vi "GetClassTemplates.vi"(0 "ClassWriterGOOP300 in":refnum<class "ClassWriterGOOP300.lvclass">, 1 "DerivedFromThisClass(if any)":refnum<vi>, 5 "error in (no error)":errorcluster) -> (14 "ClassWriterGOOP300 out":refnum<class "ClassWriterGOOP300.lvclass">, 15 "Templates":T1[](array[typedef]), 19 "error out":errorcluster)   [LabVIEW 2016, in "ClassWriterGOOP300.lvclass"]
uses:
  <resource>/Framework/Providers/Open_GDS/ClassProviders/Provider_EndevoGOOP300/ClassWriterGOOP300_class/ClassWriterGOOP300.lvclass
  <resource>/Framework/Providers/Open_GDS/ClassProviders/Provider_BaseClassInterface/ClassTemplateType.ctl
  <resource>/Framework/Providers/Open_GDS/ClassProviders/Provider_EndevoGOOP300/Templates/EndevoTemplateNames.ctl
  <resource>/Framework/Providers/Open_GDS/ClassProviders/Common/ScriptingFunctions/Scripting_ConnectorPanePatternType.ctl
  <resource>/Framework/Providers/Open_GDS/ClassProviders/Provider_BaseClassInterface/ClassWriter_class/ClassWriter.lvclass
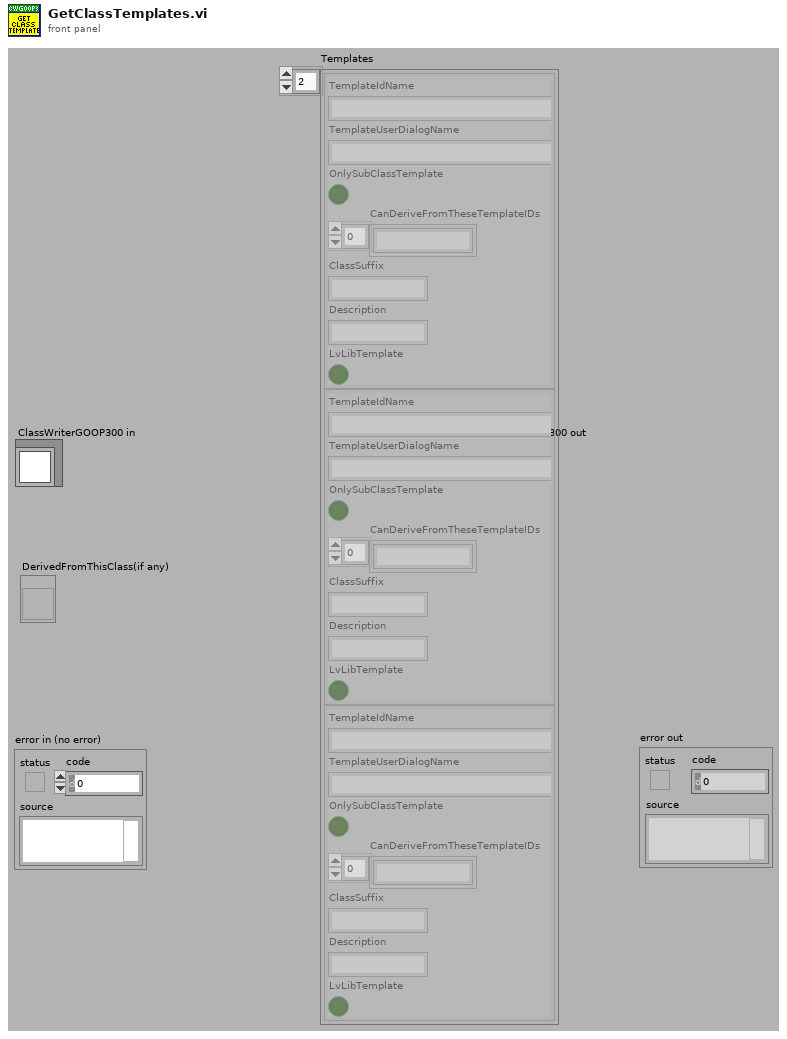
[diagram p1: front panel]
types:
  T1 = typedef "ClassWriter.lvclass/ClassTemplateType.ctl" = cluster{"TemplateIdName":string, "TemplateUserDialogName":string, "OnlySubClassTemplate":bool, "CanDeriveFromTheseTemplateIDs":string[], "ClassSuffix":string, "Description":string, "LvLibTemplate":bool}
  T2 = typedef "EndevoTemplateNames.ctl" = enum16{"BaseTemplate", "SubTemplate", "BaseTemplate_4x4x4", "SubTemplate_4x4x4", "SingletonTemplate"}
  T3 = typedef "Scripting_ConnectorPanePatternType.ctl" = u16
  T4 = typedef "GDSLvCLass_ClassSettingsType.ctl" = cluster{"ClassProviderName":string, "ClassTemplateUsed":string, "ClassTemplateVersion":string, "ClassDescription":string, "PlugIns":T5[], "ConnectorPanePattern":string}
  T5 = typedef "GDSLvClass_PlugIn.ctl" = cluster{"Type":T6, "ID":string, "Version":string, "Path":path, "Name":string, "Data":variant}
  T6 = typedef "GDSLvClass_PlugInTypes.ctl" = enum16{"DesignPattern", "MethodTypes"}
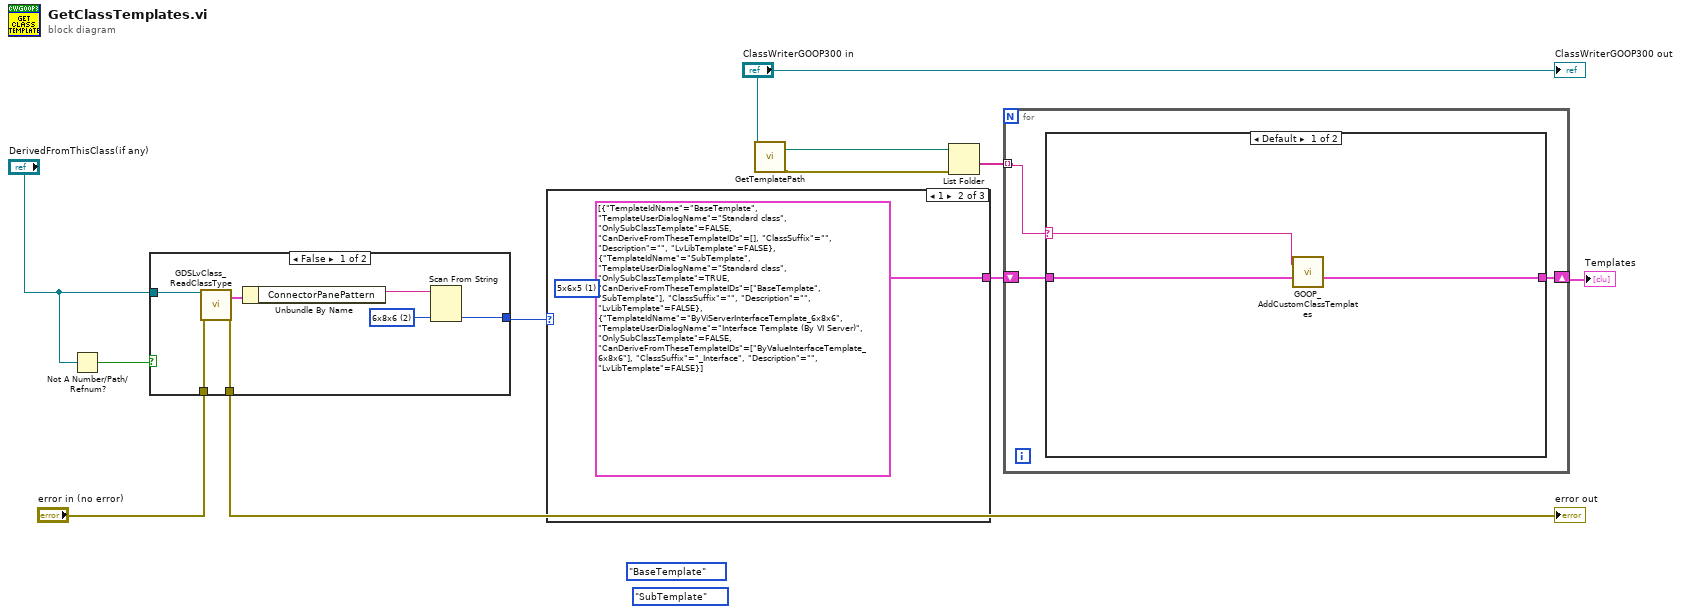
[diagram p0: block diagram]
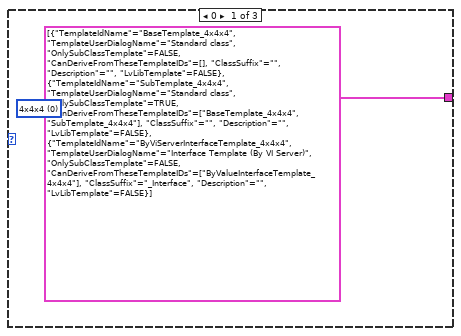
[diagram p2: hidden frame]
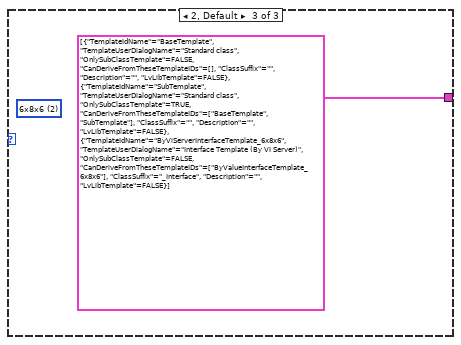
[diagram p3: hidden frame]
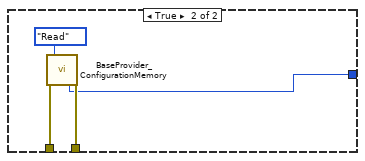
[diagram p4: hidden frame]
diagram:
  (unwired) EndevoTemplateNames."BaseTemplate" ("TemplateNames")
  (unwired) EndevoTemplateNames."SubTemplate" ("TemplateNames")
  n1 = Not A Number/Path/Refnum?(number/path/refnum="DerivedFromThisClass(if any)") -> (NaN/Path/Refnum?=w5:bool)
  n2 = case shown="False" w5 {
    tunnel: "error in (no error)" -> [w15 w21]
    tunnel: "DerivedFromThisClass(if any)" -> [w14 _]
    tunnel: [w13 w20] -> w1
    tunnel: [w12 w19] -> w4
    frame False {
      w16 = T3 2 items=["4x4x4", "5x6x5", "6x8x6"] ("Pattern")
      n3 = call <resource>:"GDSLvClass_ReadClassType.vi"("Class Refnum In"=w14, "error in (no error)"=w15) -> ("ClassSettings"=w18:T4, "error out"=w13:errorcluster)  [unwired: 15 in, 1 out]
      n4 = Unbundle By Name(w18) -> ("ConnectorPanePattern"=w17:string)
      n5 = Scan From String(input string=w17, default 1=w16) -> (output 1=w12:T3)  [unwired: 3 in, 3 out]
    }
    frame True {
      n6 = call <resource>:"BaseProvider_ConfigurationMemory.vi"("error in (no error)"=w21, "Action"=enum16{"Read", "Load", "Save"}."Read") -> ("PatternOut"=w19:T3, "error out"=w20:errorcluster)  [unwired: 11 in, 5 out]
    }
  }
  "error out" <- w1
  n7 = case shown="1" w4 {
    tunnel: [T1[] [{"TemplateIdName"="BaseTemplate_4x4x4", "TemplateUserDialogName"="Standard class", "OnlySubClassTemplate"=FALSE, "CanDeriveFromTheseTemplateIDs"=[], "ClassSuffix"="", "Description"="", "LvLibTemplate"=FALSE}, {"TemplateIdName"="SubTemplate_4x4x4", "TemplateUserDialogName"="Standard class", "OnlySubClassTemplate"=TRUE, "CanDeriveFromTheseTemplateIDs"=["BaseTemplate_4x4x4", "SubTemplate_4x4x4"], "ClassSuffix"="", "Description"="", "LvLibTemplate"=FALSE}, {"TemplateIdName"="ByViServerInterfaceTemplate_4x4x4", "TemplateUserDialogName"="Interface Template (By VI Server)", "OnlySubClassTemplate"=FALSE, "CanDeriveFromTheseTemplateIDs"=["ByValueInterfaceTemplate_4x4x4"], "ClassSuffix"="_Interface", "Description"="", "LvLibTemplate"=FALSE}] ("TemplateIdNames") T1[] [{"TemplateIdName"="BaseTemplate", "TemplateUserDialogName"="Standard class", "OnlySubClassTemplate"=FALSE, "CanDeriveFromTheseTemplateIDs"=[], "ClassSuffix"="", "Description"="", "LvLibTemplate"=FALSE}, {"TemplateIdName"="SubTemplate", "TemplateUserDialogName"="Standard class", "OnlySubClassTemplate"=TRUE, "CanDeriveFromTheseTemplateIDs"=["BaseTemplate", "SubTemplate"], "ClassSuffix"="", "Description"="", "LvLibTemplate"=FALSE}, {"TemplateIdName"="ByViServerInterfaceTemplate_6x8x6", "TemplateUserDialogName"="Interface Template (By VI Server)", "OnlySubClassTemplate"=FALSE, "CanDeriveFromTheseTemplateIDs"=["ByValueInterfaceTemplate_6x8x6"], "ClassSuffix"="_Interface", "Description"="", "LvLibTemplate"=FALSE}] ("TemplateIdNames") T1[] [{"TemplateIdName"="BaseTemplate", "TemplateUserDialogName"="Standard class", "OnlySubClassTemplate"=FALSE, "CanDeriveFromTheseTemplateIDs"=[], "ClassSuffix"="", "Description"="", "LvLibTemplate"=FALSE}, {"TemplateIdName"="SubTemplate", "TemplateUserDialogName"="Standard class", "OnlySubClassTemplate"=TRUE, "CanDeriveFromTheseTemplateIDs"=["BaseTemplate", "SubTemplate"], "ClassSuffix"="", "Description"="", "LvLibTemplate"=FALSE}, {"TemplateIdName"="ByViServerInterfaceTemplate_6x8x6", "TemplateUserDialogName"="Interface Template (By VI Server)", "OnlySubClassTemplate"=FALSE, "CanDeriveFromTheseTemplateIDs"=["ByValueInterfaceTemplate_6x8x6"], "ClassSuffix"="_Interface", "Description"="", "LvLibTemplate"=FALSE}] ("TemplateIdNames")] -> w8
    frame 0 {
      (unwired) T3 0 items=["4x4x4", "5x6x5", "6x8x6"] ("Pattern")
    }
    frame 1 {
      (unwired) T3 1 items=["4x4x4", "5x6x5", "6x8x6"] ("Pattern")
    }
    frame 2, Default {
      (unwired) T3 2 items=["4x4x4", "5x6x5", "6x8x6"] ("Pattern")
    }
  }
  n8 = call-dynamic "GetTemplatePath.vi"("reference in"="ClassWriterGOOP300 in") -> ("FolderPathOut"=w11:path, "error out"=w10:errorcluster)  [unwired: 14 in, 3 out]
  n9 = List Folder(path=w11, error in=w10) -> (folder names=w9:string[])  [unwired: 2 in, 3 out]
  n10 = for {
    tunnel: w9 -> [w26] mode=indexing
    shift-right: [w28] -> w7
    shift-left: w8 -> [w27]
    n11 = case shown="Default" w26 {
      selector: w26 -> [w31 _]
      tunnel: [w29 w32] -> w28
      tunnel: w27 -> [w30 w32]
      frame Default {
        n12 = call <resource>:"GOOP_AddCustomClassTemplates.vi"("TemplateIdNames"=w30, "String"=w31) -> ("TemplateIdNames 2"=w29:T1[])
      }
      frame "BaseTemplate", "BaseTemplate_4x4x4", "SubTemplate", "SubTemplate_4x4x4" {
      }
    }
  }
  "Templates" <- w7
  "ClassWriterGOOP300 out" <- "ClassWriterGOOP300 in"
